vi "LVClass_ModalCoef ctor Zernike From Slopes.vi"(0 "ModalCoef (const)":refnum<class "ModalCoef.lvclass">, 5 "HasoSlopes":refnum<class "HasoSlopes.lvclass">, 7 "normalization":enum16{"standard", "rms"}(ring), 9 "nb_coefs":u32, 11 "error in (no error)":errorcluster) -> (4 "ModalCoef (new)":refnum<class "ModalCoef.lvclass">, 15 "error out":errorcluster)   [LabVIEW 2020, in "ModalCoef.lvclass"]
doc: "ModalCoef constructor.\n\n--------------------------------------------------------------------------------\n\n<B>ModalCoefIn </B> : Constant Pointer to ModalCoef object.\n<B>ModalCoefOut </B> : Constant Pointer to ModalCoef object.\n<B>TypePhase </B> : TypePhase Phase mode reconstruction.\n<B>ErrorIn </B> : Error\n<B>ErrorOut </B> : Error\n\n--------------------------------------------------------------------------------"
uses:
  ModalCoef.lvclass
  HasoSlopes/HasoSlopes.lvclass
  Controls/Handle creation.ctl
  ModalCoef.lvclass/ModalCoef.ctl
  HasoSlopes/LVClass_HasoSlopes Read HasoSlopes _ property.vi
panel:
  out "HasoSlopes (dup)":refnum<class "HasoSlopes.lvclass">
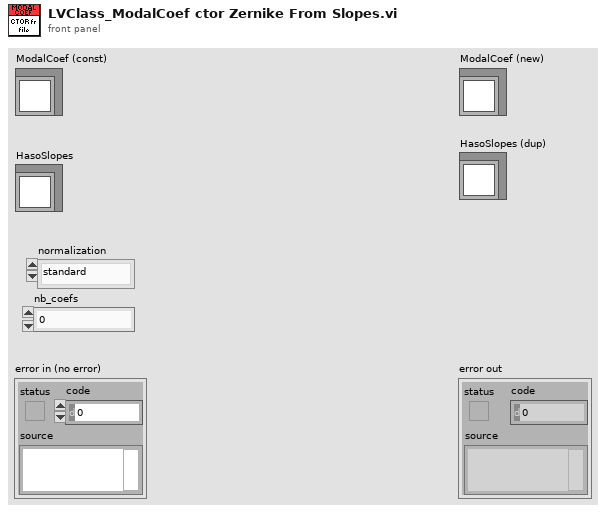
[diagram p1: front panel]
types:
  T1 = typedef "Handle creation.ctl" = enum16{"By ctor", "By write function"}
  T2 = typedef "ClassID.ctl" = i64
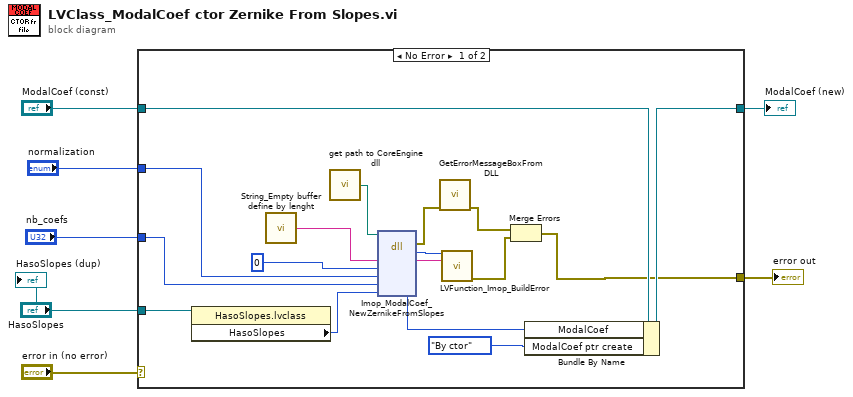
[diagram p0: block diagram]
diagram:
  n1 = case shown="No Error" "error in (no error)" {
    selector: "error in (no error)" -> [_ w26]
    tunnel: [w12 w26] -> w6
    tunnel: [w15 w25] -> w4
    tunnel: "ModalCoef (const)" -> [w16 w25]
    tunnel: "HasoSlopes" -> [w8 _]
    tunnel: "normalization" -> [w11 _]
    tunnel: "nb_coefs" -> [w10 _]
    frame No Error {
      n2 = property class="HasoSlopes.lvclass"(reference=w8) -> ("HasoSlopes"=w9:T2)  [unwired: 1 in, 2 out]
      n3 = call "String_Empty buffer define by lenght.vi"() -> ("Empty buffer"=w24:string)  [unwired: 1 in]
      n4 = call "get path to CoreEngine dll.vi"() -> ("path to wavekit library"=w21:path)  [unwired: 14 in, 1 out]
      n5 = dll-call lib="D:/soft/HASO_v3/SVN_trunk/ImOpCoreEngine4_LV2011/DLLs/c_interface_vc100.dll" fn="Imop_ModalCoef_NewZernikeFromSlopes"(path in=w21, "message"=w24, "ModalCoef"=0 ("Pupil"), "Normalization"=w11, "nb_coefs"=w10, "Slopes"=w9) -> (error out=w20:errorcluster, "return type"=w22:i32, "message"=w23:string, "ModalCoef"=w18:i64)  [unwired: 5 in, 1 out]
      n6 = call "GetErrorMessageBoxFromDLL.vi"("error IN"=w20) -> ("error OUT"=w14:errorcluster)  [unwired: 10 in]
      n7 = call "LVFunction_Imop_BuildError.vi"("code"=w22, "String to Prepend to source (\"\")"=w23) -> ("error out"=w13:errorcluster)  [unwired: 13 in]
      n8 = Merge Errors(w14, w13) -> (w12:errorcluster)
      n9 = Bundle By Name(cluster=w16, "ModalCoef"=w18, "ModalCoef ptr create"=Handle_creation."By ctor" ("Pupil ptr create")) -> (w15:refnum<class "ModalCoef.lvclass">)
    }
    frame Error {
    }
  }
  "error out" <- w6
  "ModalCoef (new)" <- w4
  "HasoSlopes (dup)" <- "HasoSlopes"
